vi "Array_Investigation part 3.vi"() -> ()   [LabVIEW 2014]
doc: "This VI is an exercise in the LabVIEW Core I course.\n\nEnter the number of columns and rows you want generated, then run the VI. This VI generates an array with the number of rows and columns you specify."
panel:
  out "second column":dbl[](array[numeric])
  out "third row":dbl[](array[numeric])
  out "Intensity Graph":dbl[][](graph)
  out "Array":dbl[][](array[numeric])
  in  "Rows":i32=80
  in  "Columns":i32=80
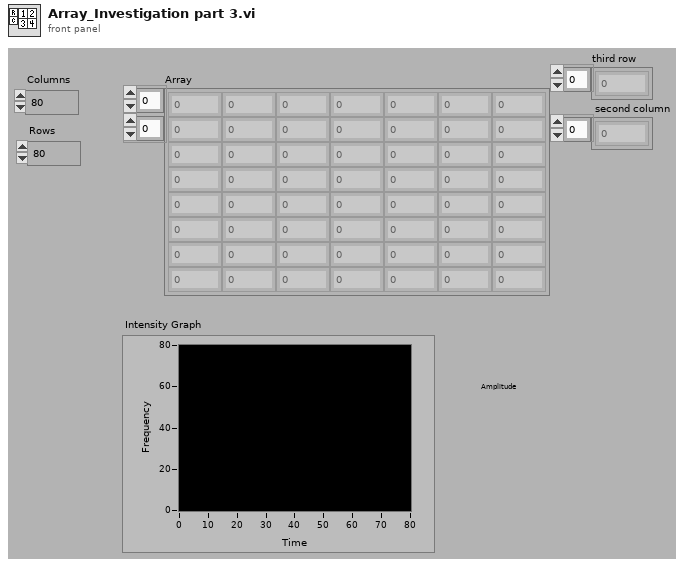
[diagram p1: front panel]
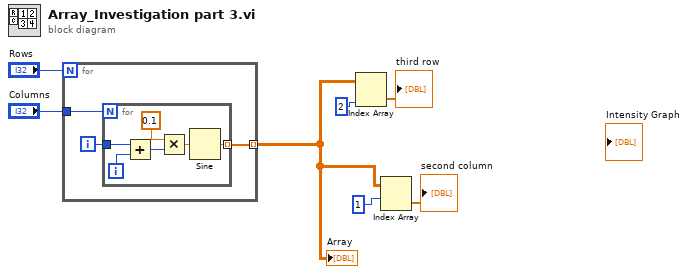
[diagram p0: block diagram]
diagram:
  n1 = for {
    N: "Rows" -> [_]
    tunnel: [w10] -> w5 mode=indexing
    tunnel: "Columns" -> [w9]
    i -> [w8]
    n2 = for {
      N: w9 -> [_]
      tunnel: [w16] -> w10 mode=indexing
      tunnel: w8 -> [w13]
      i -> [w14]
      n3 = Add(x=w13, y=w14) -> (x+y=w15:i32)
      n4 = Multiply(x=0.1, y=w15) -> (x*y=w12:dbl)
      n5 = Sine(x=w12) -> (sin(x)=w16:dbl)
    }
  }
  "Array" <- w5
  n6 = Index Array(array=w5, index (col)=2) -> (element=→"third row":dbl[])  [unwired: 1 in]
  n7 = Index Array(array=w5, index (row)=1) -> (element=→"second column":dbl[])  [unwired: 1 in]
